vi "Replace Temp Thresholds.vi"(6 "Cal Abort Threshold (R/4)":string="NaN", 8 "Cal Critical Threshold (R/4)":string="NaN", 9 "Cal Warning Threshold (R/4)":string="NaN", 10 "Cal Minimum Threshold (R/4)":string="NaN", 11 "Gen Cals In":string="Reserved[00]=0x00\nReserved[01]=0x00\nReserved[02]=0x00\nReserved[03]=0x00\nReserved[04]=0x00\nReserved[05]=0x00\nReserved[06]=0x00\nReserved[07]=0x00\nReserved[08]=0x00\t\t\nReserved[09]=0x00\nReserved[10]=0x00\nReserved[11]=0x00\nReserved[12]=0x00\nReserved[13]=0x00\nReserved[14]=0x00\ntempMinThreshold=0xCAC4\ntempWarningThresholdl=0x31D3\ntempCriticalThresholdl=0x2FBB\ntempAbortThresholdl=0x2DBD\nthermOffsetMinimum=0x190\nthermOffsetMaximum=0x320\nthermBiasMinimum=0x3E8\nthermBiasMaximum=0xD48\nthermInputMinimum=0x384\nthermInputMaximum=0xC1C\nbatteryIncreasePreCharge=0x19\nbatteryIncreaseConstandCurrent=0x08\nReserved[00]=0x00\nReserved[01]=0x00\nReserved[02]=0x00\nReserved[03]=0x00\nReserved[04]=0x00\nReserved[05]=0x00\nReserved[06]=0x00\nReserved[07]=0x00\nReserved[08]=0x00\nReserved[09]=0x00\nReserved[10]=0x00\nReserved[11]=0x00\nReserved[12]=0x00\nReserved[13]=0x00\nReserved[14]=0x00\nbatteryStateCalStimOff[00]=0xCDE\nbatteryStateCalStimOff[01]=0xC8B\nbatteryStateCalStimOff[02]=0xC4F\nbatteryStateCalStimOff[03]=0xC2E\nbatteryStateCalStimOff[04]=0xC0C\nbatteryStateCalStimOff[05]=0x948\nbatteryStateCalStimOn[00]=0xCCB\nbatteryStateCalStimOn[01]=0xC75\nbatteryStateCalStimOn[02]=0xC3B\nbatteryStateCalStimOn[03]=0xC19\nbatteryStateCalStimOn[04]=0xBFC\nbatteryStateCalStimOn[05]=0x948\nvrectMeasurementCal=0x2EE") -> (3 "Gen Cals Out":string)   [LabVIEW 2010]
doc: "This function parses an IPG Temperature Threshold Status string into four Resistance values.\n\nIf the status string format is incorrect, <not available> and NaN values will be returned."
panel:
  # "Temperature thresholds\nin hex multiplied by four."
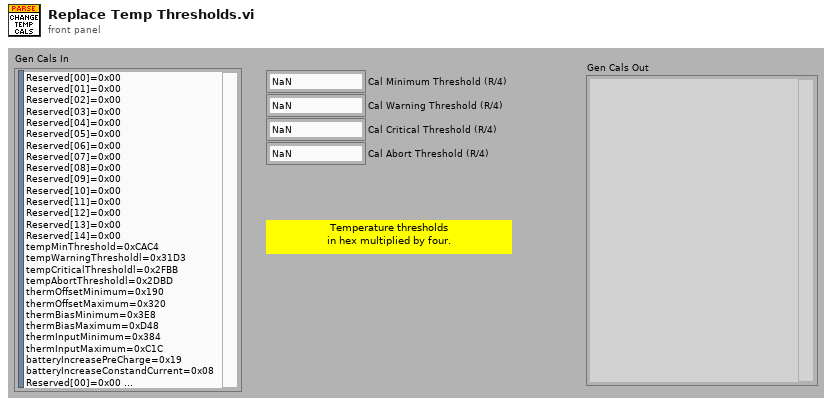
[diagram p1: front panel]
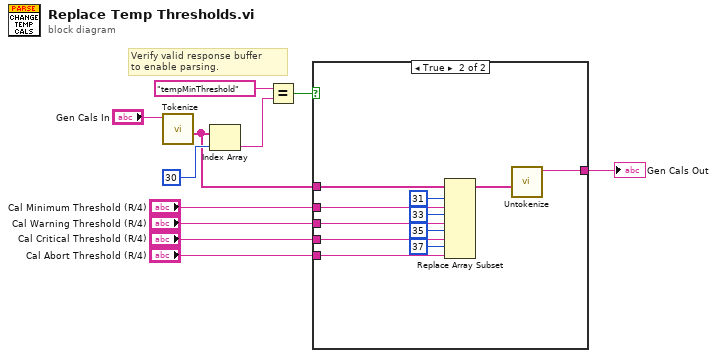
[diagram p0: block diagram]
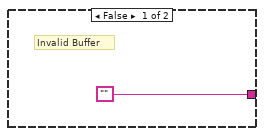
[diagram p2: hidden frame]
diagram:
  # "Verify valid response buffer\nto enable parsing."
  n1 = call "Tokenize.vi"("input string"="Gen Cals In") -> ("tokens"=w2:string[])  [unwired: 4 in, 2 out]
  n2 = Index Array(array=w2, index=30) -> (element=w3:string)
  n3 = Equal?(x="tempMinThreshold", y=w3) -> (x = y?=w10:bool)
  n4 = case shown="True" w10 {
    tunnel: "Cal Minimum Threshold (R/4)" -> [_ w19]
    tunnel: "Cal Warning Threshold (R/4)" -> [_ w18]
    tunnel: "Cal Critical Threshold (R/4)" -> [_ w17]
    tunnel: "Cal Abort Threshold (R/4)" -> [_ w16]
    tunnel: w2 -> [_ w15]
    tunnel: ["" w13] -> w1
    frame False {
      # "Invalid Buffer"
    }
    frame True {
      n5 = Replace Array Subset(array=w15, new element #1=w19, index #1=31 ("index"), new element #2=w18, index #2=33 ("index"), new element #3=w17, index #3=35 ("index"), new element #4=w16, index #4=37 ("index")) -> (w14:string[])
      n6 = call "Untokenize.vi"("tokens"=w14) -> ("string out"=w13:string)  [unwired: 10 in]
    }
  }
  "Gen Cals Out" <- w1
